vi "Get Sequencer DVR.vi"(8 "Error In":errorcluster, 11 "Sequencer In":refnum<class "Sequencer.lvclass">) -> (0 "Error Out":errorcluster, 2 "DVR":refnum<data-value>, 3 "Sequencer Out":refnum<class "Sequencer.lvclass">)   [LabVIEW 2019, in "Sequencer.lvclass"]
uses:
  Sequencer.lvclass
  Controls/Data.ctl
  Sequencer.lvclass/Sequencer.ctl
  Utilities/Utilities.lvlib
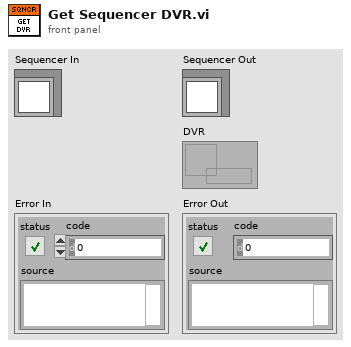
[diagram p1: front panel]
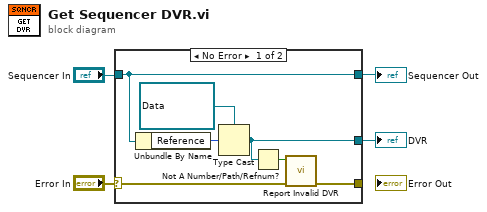
[diagram p0: block diagram]
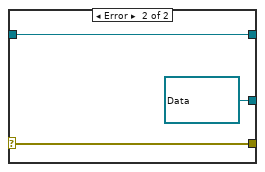
[diagram p2: hidden frame]
diagram:
  n1 = case shown="No Error" "Error In" {
    selector: "Error In" -> [w6 w14]
    tunnel: "Sequencer In" -> [w10 w13]
    tunnel: [w5 w14] -> _
    tunnel: [w10 w13] -> w2
    tunnel: [w8 refnum<data-value> refnum ("data value reference")] -> w1
    frame No Error {
      n2 = Unbundle By Name(w10) -> ("Reference"=w11:u64)
      n3 = Type Cast(type=refnum<data-value> refnum ("data value reference"), x=w11) -> (*(type *) &x=w8:refnum<data-value>)
      n4 = Not A Number/Path/Refnum?(number/path/refnum=w8) -> (NaN/Path/Refnum?=w7:bool)
      n5 = call "Report Invalid DVR.vi"("Error In"=w6, "Invalid DVR"=w7) -> ("Error Out"=w5:errorcluster)  [unwired: 9 in]
    }
    frame Error {
    }
  }
  "Sequencer Out" <- w2
  "DVR" <- w1
